vi "Main.vi"(11 "Module Admin":refnum<class "Delacor_lib_QMH_Module Admin.lvclass">) -> ()   [LabVIEW 2020, in "Settings.lvlib"]
doc: "This template is based off of the Queued Message Handler design pattern and the Queued Message Handler project template that ships with LabVIEW.\n\nThe main difference is that the queue is private to this module and communication between modules is performed via Broadcast and Request events.\n\nRequest events are wrapped in public API methods and are handled in the Event Handling Loop (EHL) of this VI. Any module can register for Broadcast events sent by this module. The EHL generates messages based on user interface actions.\n\nThe Message Handling Loop (MHL) processes messages generated by the EHL, or by other messages. The messages are string values, so new messages can be added easily to the Message Cases case structure in the MHL. Each message cluster can also provide an optional value for Message Data, which is a variant that can be converted to whatever message-specific data is required.\n_____\nBased on Delacor QMH Project Template 6.0.0.89."
uses:
  Settings.lvlib
  <vilib>/Delacor/Delacor QMH/Libraries/Module Admin_class/Delacor_lib_QMH_Module Admin.lvclass
  typeSignal--cluster.ctl
  Module Data--cluster.ctl
  Stop Argument--cluster.ctl
  <vilib>/Delacor/Delacor QMH/Libraries/Message Queue_class/Delacor_lib_QMH_Message Queue.lvclass/Delacor_lib_QMH_Message Queue.ctl
  <vilib>/Delacor/Delacor QMH/Libraries/Module Admin_class/Delacor_lib_QMH_Module Admin.lvclass/Delacor_lib_QMH_Module Admin.ctl
  Add signal Argument--cluster.ctl
  Add Digital Signal Argument--cluster.ctl
  Complete Tarea Argument--cluster.ctl
  Delete table Argument--cluster.ctl
  Delete Digital table Argument--cluster.ctl
  Delete All Table Argument--cluster.ctl
  Cancel Argument--cluster.ctl
  Type Signal loaded form database Argument--cluster.ctl
  <vilib>/Utility/miscctls.llb/LVPointTypeDef.ctl
  <vilib>/Delacor/Delacor QMH/Libraries/Message Queue_class/Delacor_lib_QMH_Enqueue Message (Single).vi
  <vilib>/Delacor/Delacor QMH/Libraries/Module Admin_class/Delacor_lib_QMH_Get External Launch.vi
  <vilib>/Utility/error.llb/Error Cluster From Error Code.vi
  <vilib>/ErrorRing/Error Ring.xnode
  <vilib>/Delacor/Delacor QMH/Libraries/Message Queue_class/Delacor_lib_QMH_Message Queue.lvclass
panel:
  in  "Tarea Lista":bool
  in  "Tab Control":enum32{"Page 1", "Page 2"}(tab)
  in  "Agregar Tarea":bool
  in  "Borrar una Tarea":bool
  in  "Analog Signal":T1={"DAQ Board Name"="DAQ_Simu1", "Analogicos Canales"=["DAQ_Simu1/ai1", "DAQ_Simu1/ai2"], "Port Digitales"=[], "Tiempo"=100.0, "number of samples "=1000, "rate"=1000.0, "Type"=enum."Analogico"}
  in  "Digital Signal":T1={"DAQ Board Name"="DAQ_Simu1", "Analogicos Canales"=["DAQ_Simu1/ai1", "DAQ_Simu1/ai2"], "Port Digitales"=[], "Tiempo"=100.0, "number of samples "=1000, "rate"=1000.0, "Type"=enum."Analogico"}
  in  "Borrar una Tarea Digital":bool
  in  "Agregar Tarea Digital":bool
  in  "Borrar todo":bool
  in  "Cancel Button":bool
  in  "Nombre de la Prueba":string
  out "error out":errorcluster
  out "Status":string
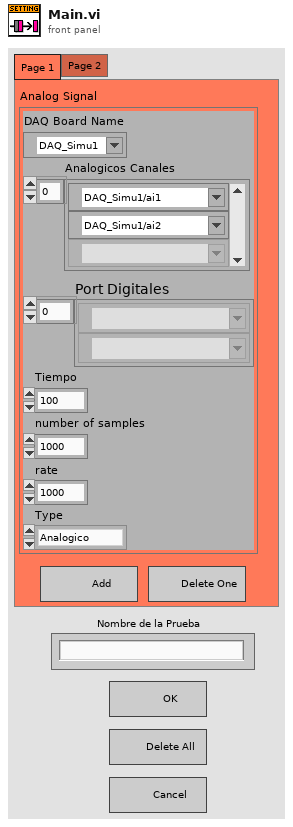
[diagram p1: front panel]
types:
  T1 = typedef "typeSignal--cluster.ctl" = cluster{"DAQ Board Name":tag, "Analogicos Canales":tag[], "Port Digitales":tag[], "Tiempo":dbl, "number of samples ":i32, "rate":dbl, "Type":enum16{"Analogico", "Digital"}}
  T2 = typedef "Settings.lvlib/Request Events--cluster.ctl" = cluster{"Stop Module":refnum<user-event>, "Show Panel":refnum<user-event>, "Hide Panel":refnum<user-event>, "Get Module Execution Status":refnum<user-event>, "Show Diagram":refnum<user-event>, "Add signal":refnum<user-event>, "Delete table":refnum<user-event>, "Cancel":refnum<user-event>, "Type Signal loaded form database":refnum<user-event>, "Delete All Table":refnum<user-event>, "Add Digital Signal":refnum<user-event>, "Delete Digital table":refnum<user-event>, "Complete Tarea":refnum<user-event>}
  T3 = typedef "Settings.lvlib/Module Data--cluster.ctl" = cluster{"Status":string, "Type Signal":T1, "Nombre de la Prueba":string}
  T4 = enum32{"invalid lock state", "Not Locked", "Locked (No Password)", "Password-protected"}
  T5 = typedef "Settings.lvlib/Stop Argument--cluster.ctl" = cluster{"Origin":string, "Exit via Stop Module Req?":bool, "Wait for Module to stop?":bool}
  T6 = typedef "Settings.lvlib/Add signal Argument--cluster.ctl" = cluster{"Agregar Tarea":bool}
  T7 = typedef "Settings.lvlib/Add Digital Signal Argument--cluster.ctl" = cluster{"Agregar Tarea Digital":bool}
  T8 = typedef "Settings.lvlib/Complete Tarea Argument--cluster.ctl" = cluster{"Tarea Lista":bool}
  T9 = typedef "Settings.lvlib/Delete table Argument--cluster.ctl" = cluster{"Borrar Tarea":bool}
  T10 = typedef "Settings.lvlib/Delete Digital table Argument--cluster.ctl" = cluster{"Borrar una Tarea Digital":bool}
  T11 = typedef "Settings.lvlib/Delete All Table Argument--cluster.ctl" = cluster{"Borrar todo":bool}
  T12 = typedef "Settings.lvlib/Cancel Argument--cluster.ctl" = cluster{"Cancel Button":bool}
  T13 = typedef "Settings.lvlib/Type Signal loaded form database Argument--cluster.ctl" = cluster{"Type Signal":T1, "Nombre de la Prueba":string}
  T14 = typedef "LVPointTypeDef.ctl" = cluster{"Horizontal":i16, "Vertical":i16}
  T15 = enum32{"Invalid", "Standard", "Closed", "Hidden", "Minimized", "Maximized"}
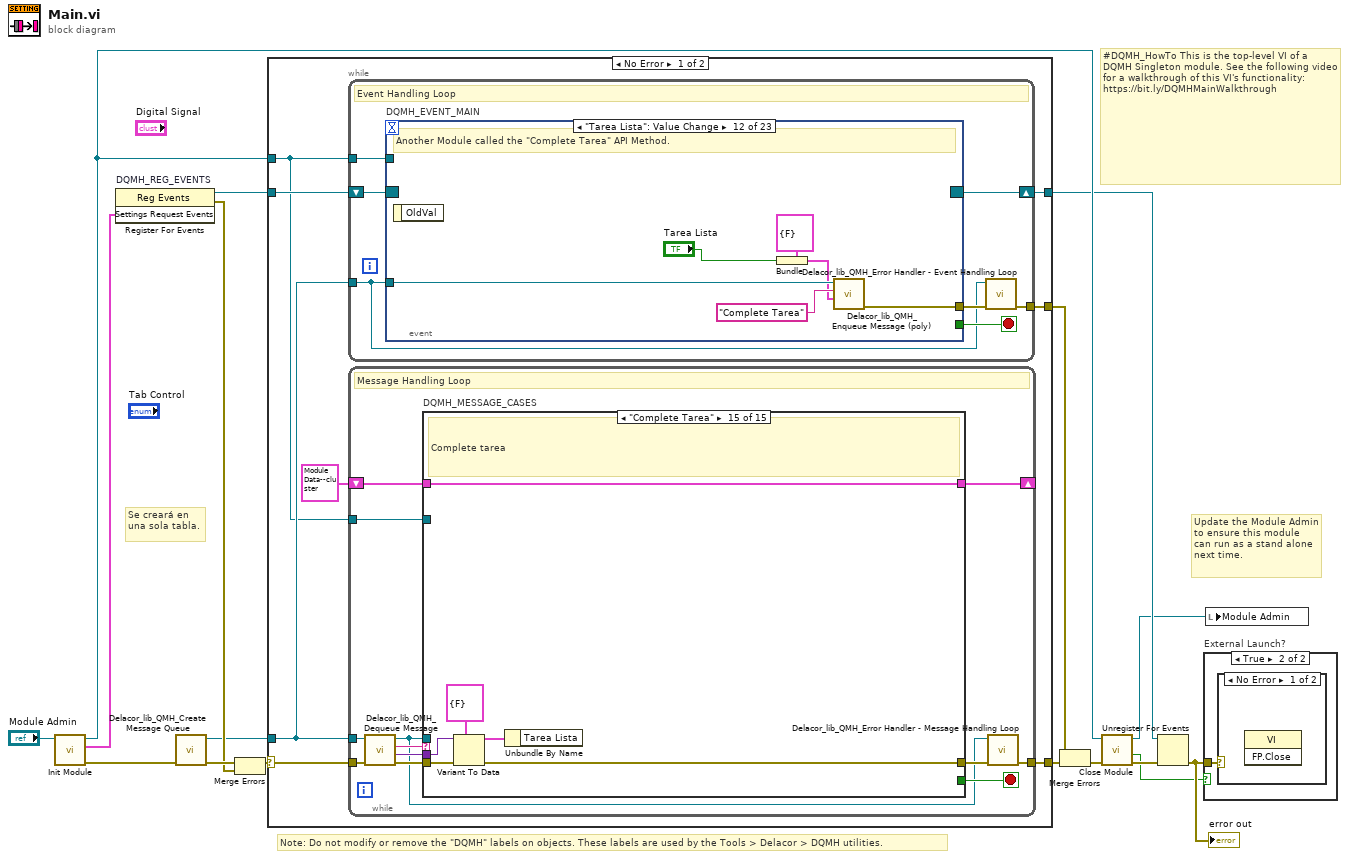
[diagram p0: block diagram]
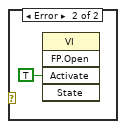
[diagram p3: hidden frame]
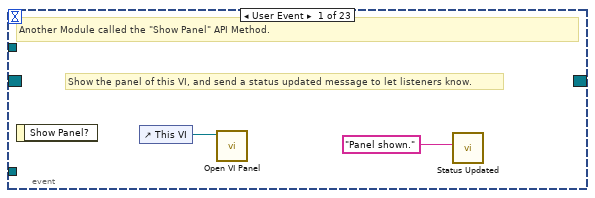
[diagram p4: hidden frame]
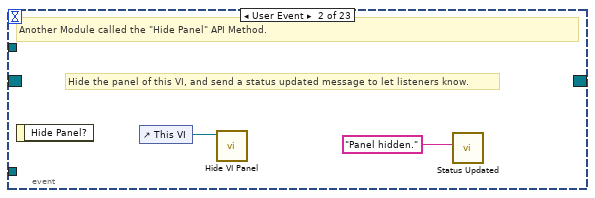
[diagram p5: hidden frame]
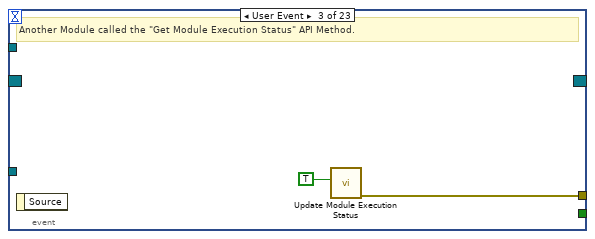
[diagram p6: hidden frame]
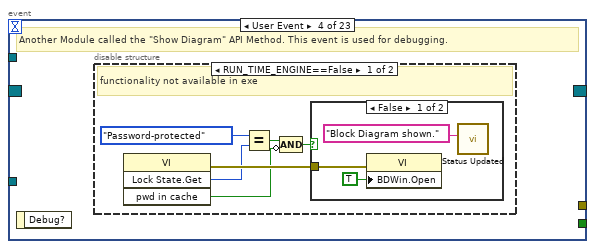
[diagram p7: hidden frame]
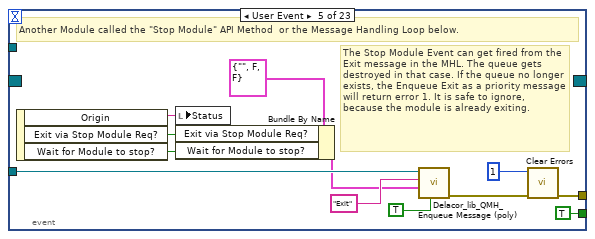
[diagram p10: hidden frame]
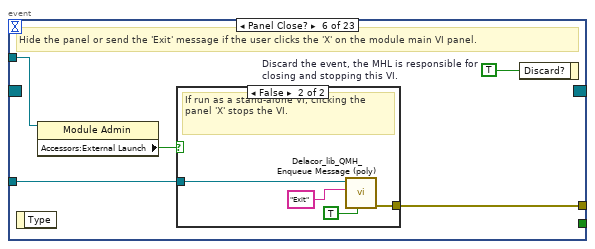
[diagram p11: hidden frame]
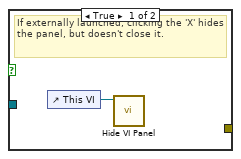
[diagram p12: hidden frame]
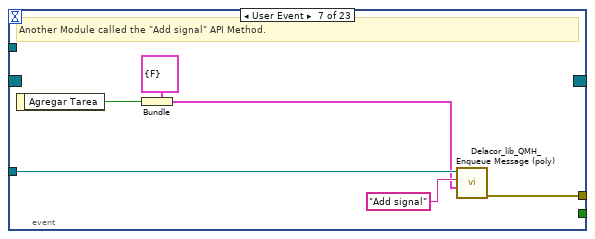
[diagram p13: hidden frame]
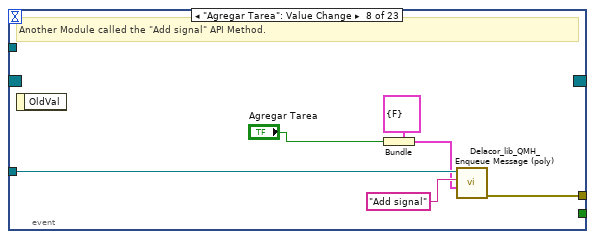
[diagram p14: hidden frame]
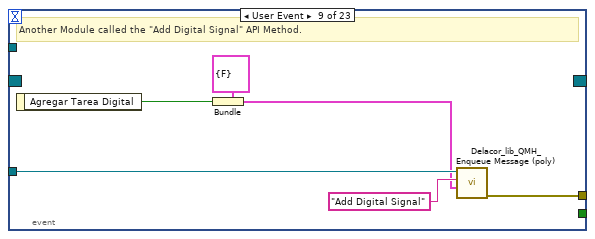
[diagram p15: hidden frame]
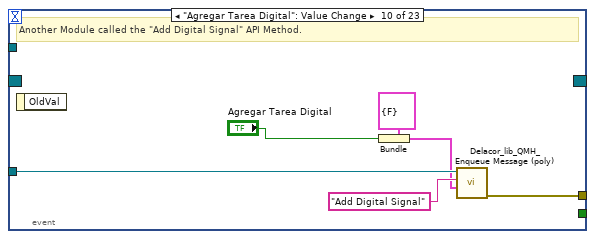
[diagram p16: hidden frame]
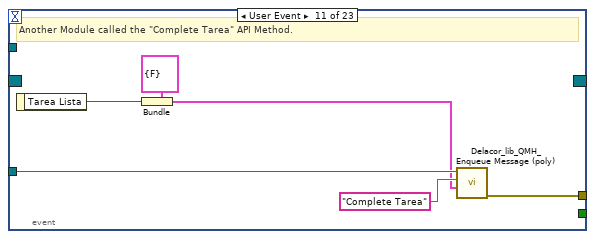
[diagram p17: hidden frame]
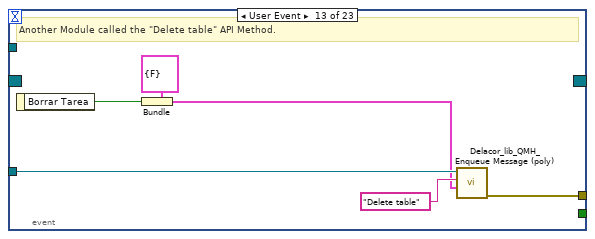
[diagram p18: hidden frame]
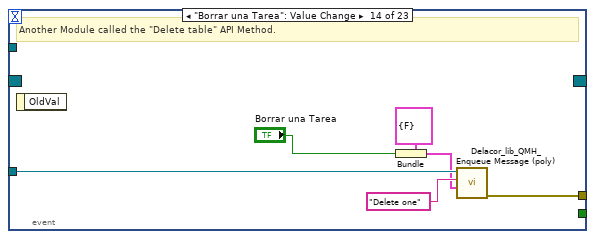
[diagram p19: hidden frame]
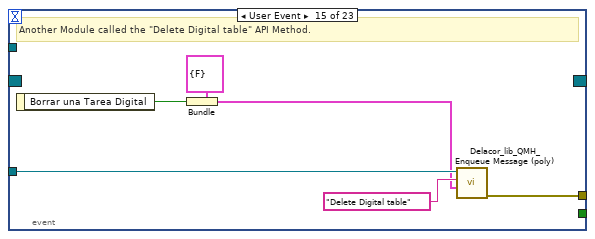
[diagram p20: hidden frame]
diagram:
  # "Se creará en una sola tabla."
  # "#DQMH_HowTo This is the top-level VI of a DQMH Singleton module. See the following video for a walkthrough of this VI's functionality: https://bit.ly/DQMHMainWalkthrough"
  # "Note: Do not modify or remove the \"DQMH\" labels on objects. These labels are used by the Tools > Delacor > DQMH utilities."
  # "Update the Module Admin to ensure this module can run as a stand alone next time."
  n1 = call "Init Module.vi"("Singleton Module Admin in"="Module Admin") -> ("error out"=w16:errorcluster, "Settings Request Events"=w5:T2, "Singleton Module Admin out"=w8:refnum<class "Delacor_lib_QMH_Module Admin.lvclass">)  [unwired: 8 in]
  n2 = register-events "DQMH_REG_EVENTS"(w5) -> (reference out=w6:refnum<event-registration>, error out=w9:errorcluster)  [unwired: 2 in]
  n3 = call <vilib>:"Delacor_lib_QMH_Create Message Queue.vi"("error in"=w16) -> ("error out"=w11:errorcluster, "Message Queue"=w4:refnum<class "Delacor_lib_QMH_Message Queue.lvclass">)  [unwired: 9 in]
  n4 = Merge Errors(w11, w9) -> (w10:errorcluster)
  n5 = case shown="No Error" w10 {
    selector: w10 -> [w23 w343]
    tunnel: [w25 w342] -> w17
    tunnel: [w22 w348] -> w7
    tunnel: w6 -> [w20 w348]
    tunnel: w4 -> [w19 w341]
    tunnel: [w24 _] -> w14
    tunnel: w8 -> [w18 w344]
    frame No Error {
      n6 = while {
        tunnel: w19 -> [w26]
        shift-right: [w29] -> w22
        shift-left: w20 -> [w30]
        tunnel: [w31] -> w24
        tunnel: w18 -> [w27]
        stop <- w28 stop-if-true
        # "Event Handling Loop"
        n7 = event "DQMH_EVENT_MAIN" shown="[11] \"Tarea Lista\": Value Change" {
          selector: w30 -> [_ _ _ _ _ _ _ _ _ _ _ _ _ _ _ _ _ _ _ _ _ _ _]
          dyn-events: [_ _ _ _ _ _ _ _ _ _ _ _ _ _ _ _ _ _ _ _ _ _ _] -> w29
          timeout: _ -> [_ _ _ _ _ _ _ _ _ _ _ _ _ _ _ _ _ _ _ _ _ _ _]
          tunnel: [_ _ _ _ TRUE ("Discard?") _ _ _ _ _ _ _ _ _ _ _ _ _ _ _ _ _ _] -> w28
          tunnel: w26 -> [_ _ _ _ w55 w62 w75 w81 w87 w93 w99 w105 w111 w117 w123 w129 w135 w141 w147 w153 w157 w161 w168]
          tunnel: [_ _ w38 _ w58 w64 w70 w77 w82 w89 w94 w101 w106 w113 w118 w125 w130 w137 w142 w149 w156 w160 w162] -> w32
          tunnel: w27 -> [_ _ _ _ _ w61 _ _ _ _ _ _ _ _ _ _ _ _ _ _ _ _ _]
          event User Event {
            # "Show the panel of this VI, and send a status updated message to let listeners know."
            # "Another Module called the \"Show Panel\" API Method."
            n8 = event-data() -> ()  [unwired: 1 in, 1 out]
            n9 = control-ref of="This VI"() -> (w34:refnum<vi>)
            n10 = call "Open VI Panel.vi"("VI"=w34) -> ()  [unwired: 10 in, 1 out]
            n11 = call "Status Updated.vi"("Status"="Panel shown." ("format string")) -> ()  [unwired: 10 in, 1 out]
          }
          event User Event {
            # "Hide the panel of this VI, and send a status updated message to let listeners know."
            # "Another Module called the \"Hide Panel\" API Method."
            n12 = event-data() -> ()  [unwired: 1 in, 1 out]
            n13 = control-ref of="This VI"() -> (w36:refnum<vi>)
            n14 = call "Hide VI Panel.vi"("VI"=w36) -> ()  [unwired: 10 in, 1 out]
            n15 = call "Status Updated.vi"("Status"="Panel hidden." ("format string")) -> ()  [unwired: 10 in, 1 out]
          }
          event User Event {
            # "Another Module called the \"Get Module Execution Status\" API Method."
            n16 = event-data() -> ()  [unwired: 1 in, 1 out]
            n17 = call "Update Module Execution Status.vi"("Running?"=TRUE) -> ("error out"=w38:errorcluster)  [unwired: 10 in]
          }
          event User Event {
            # "Another Module called the \"Show Diagram\" API Method. This event is used for debugging."
            n18 = event-data() -> ()  [unwired: 1 in, 1 out]
            n19 = disable-structure shown="RUN_TIME_ENGINE==False" {
              frame condition #0 (active) {
                # "functionality not available in exe"
                n20 = invoke class="VI" method="Lock State.Get"() -> (error out=w44:errorcluster, "Get Lock State"=w43:T4, "pwd in cache"=w40:bool)  [unwired: 4 in, 1 out]
                n21 = Equal?(x=T4."Password-protected", y=w43) -> (x = y?=w41:bool)
                n22 = Compound Arithmetic op=AND(w41, invert w40) -> (w39:bool)
                n23 = case shown="False" w39 {
                  tunnel: w44 -> [w47 _]
                  frame False {
                    n24 = property class="VI"(error in=w47, "BDWin.Open"=TRUE ("Block Diagram Window:Open")) -> ()  [unwired: 1 in, 2 out]
                    n25 = call "Status Updated.vi"("Status"="Block Diagram shown." ("format string")) -> ()  [unwired: 10 in, 1 out]
                  }
                  frame True {
                    # "Password-protected VI, and the password is not in the cache. Do not show the diagram."
                  }
                }
              }
              frame condition #1 {
              }
            }
          }
          event User Event {
            # "The Stop Module Event can get fired from the Exit message in the MHL. The queue gets destroyed in that case. If the queue no longer exists, the Enqueue Exit as a priority message will return error 1. It is safe to ignore, because the module is already exiting."
            # "Another Module called the \"Stop Module\" API Method  or the Message Handling Loop below."
            n26 = event-data() -> ("Origin"=w54:string, "Exit via Stop Module Req?"=w50:bool, "Wait for Module to stop?"=w49:bool)  [unwired: 1 in]
            n27 = local write "Status"(w54) -> ()
            n28 = Bundle By Name(cluster=T5 {"Origin"="", "Exit via Stop Module Req?"=FALSE, "Wait for Module to stop?"=FALSE} ("Stop Argument"), "Exit via Stop Module Req?"=w50, "Wait for Module to stop?"=w49) -> (w48:T5)
            n29 = call-poly <vilib>:"Delacor_lib_QMH_Enqueue Message (poly).vi"("Priority Message? (F)"=TRUE, "Message Data"=w48, "Message"="Exit", "Message Queue in"=w55) -> ("error out"=w59:errorcluster)  [unwired: 6 in, 1 out]
            n30 = call <vilib>:"Clear Errors.vi"("error in (no error)"=w59, "specific error code to clear (0: all)"=1) -> ("error out"=w58:errorcluster)  [unwired: 4 in, 1 out]
          }
          event Panel Close? {
            w63 = TRUE  # Discard the event, the MHL is responsible for closing and stopping this VI.
            # "Hide the panel or send the 'Exit' message if the user clicks the 'X' on the module main VI panel."
            n31 = event-data() -> ()  [unwired: 1 in, 1 out]
            n32 = property class="Module Admin"(reference=w61) -> ("Accessors:External Launch"=w60:bool)  [unwired: 1 in, 2 out]
            n33 = case shown="False" w60 {
              tunnel: w62 -> [_ w68]
              tunnel: [_ w69] -> w64
              frame True {
                # "If externally launched, clicking the 'X' hides the panel, but doesn't close it."
                n34 = control-ref of="This VI"() -> (w65:refnum<vi>)
                n35 = call "Hide VI Panel.vi"("VI"=w65) -> ()  [unwired: 10 in, 1 out]
              }
              frame False {
                # "If run as a stand-alone VI, clicking the panel 'X' stops the VI."
                n36 = call-poly <vilib>:"Delacor_lib_QMH_Enqueue Message (poly).vi"("Priority Message? (F)"=TRUE, "Message"="Exit", "Message Queue in"=w68) -> ("error out"=w69:errorcluster)  [unwired: 7 in, 1 out]
              }
            }
            n37 = event-data("Discard?"=w63) -> ()  [unwired: 1 in, 1 out]
          }
          event User Event {
            # "Another Module called the \"Add signal\" API Method."
            n38 = event-data() -> ("Agregar Tarea"=w71:bool)  [unwired: 1 in]
            n39 = Bundle(cluster=T6 {"Agregar Tarea"=FALSE} ("Add signal Argument"), "Agregar Tarea"=w71) -> (w72:T6)
            n40 = call-poly <vilib>:"Delacor_lib_QMH_Enqueue Message (poly).vi"("Message Data"=w72, "Message"="Add signal", "Message Queue in"=w75) -> ("error out"=w70:errorcluster)  [unwired: 7 in, 1 out]
          }
          event "Agregar Tarea": Value Change {
            # "Another Module called the \"Add signal\" API Method."
            n41 = event-data() -> ()  [unwired: 1 in, 1 out]
            n42 = Bundle(cluster=T6 {"Agregar Tarea"=FALSE} ("Add signal Argument"), "Agregar Tarea"="Agregar Tarea") -> (w78:T6)
            n43 = call-poly <vilib>:"Delacor_lib_QMH_Enqueue Message (poly).vi"("Message Data"=w78, "Message"="Add signal", "Message Queue in"=w81) -> ("error out"=w77:errorcluster)  [unwired: 7 in, 1 out]
          }
          event User Event {
            # "Another Module called the \"Add Digital Signal\" API Method."
            n44 = event-data() -> ("Agregar Tarea Digital"=w83:bool)  [unwired: 1 in]
            n45 = Bundle(cluster=T7 {"Agregar Tarea Digital"=FALSE} ("Add Digital Signal Argument"), "Agregar Tarea Digital"=w83) -> (w84:T7)
            n46 = call-poly <vilib>:"Delacor_lib_QMH_Enqueue Message (poly).vi"("Message Data"=w84, "Message"="Add Digital Signal", "Message Queue in"=w87) -> ("error out"=w82:errorcluster)  [unwired: 7 in, 1 out]
          }
          event "Agregar Tarea Digital": Value Change {
            # "Another Module called the \"Add Digital Signal\" API Method."
            n47 = event-data() -> ()  [unwired: 1 in, 1 out]
            n48 = Bundle(cluster=T7 {"Agregar Tarea Digital"=FALSE} ("Add Digital Signal Argument"), "Agregar Tarea Digital"="Agregar Tarea Digital") -> (w90:T7)
            n49 = call-poly <vilib>:"Delacor_lib_QMH_Enqueue Message (poly).vi"("Message Data"=w90, "Message"="Add Digital Signal", "Message Queue in"=w93) -> ("error out"=w89:errorcluster)  [unwired: 7 in, 1 out]
          }
          event User Event {
            # "Another Module called the \"Complete Tarea\" API Method."
            n50 = event-data() -> ("Tarea Lista"=w95:bool)  [unwired: 1 in]
            n51 = Bundle(cluster=T8 {"Tarea Lista"=FALSE} ("Complete Tarea Argument"), "Tarea Lista"=w95) -> (w96:T8)
            n52 = call-poly <vilib>:"Delacor_lib_QMH_Enqueue Message (poly).vi"("Message Data"=w96, "Message"="Complete Tarea", "Message Queue in"=w99) -> ("error out"=w94:errorcluster)  [unwired: 7 in, 1 out]
          }
          event "Tarea Lista": Value Change {
            # "Another Module called the \"Complete Tarea\" API Method."
            n53 = event-data() -> ()  [unwired: 1 in, 1 out]
            n54 = Bundle(cluster=T8 {"Tarea Lista"=FALSE} ("Complete Tarea Argument"), "Tarea Lista"="Tarea Lista") -> (w102:T8)
            n55 = call-poly <vilib>:"Delacor_lib_QMH_Enqueue Message (poly).vi"("Message Data"=w102, "Message"="Complete Tarea", "Message Queue in"=w105) -> ("error out"=w101:errorcluster)  [unwired: 7 in, 1 out]
          }
          event User Event {
            # "Another Module called the \"Delete table\" API Method."
            n56 = event-data() -> ("Borrar Tarea"=w107:bool)  [unwired: 1 in]
            n57 = Bundle(cluster=T9 {"Borrar Tarea"=FALSE} ("Delete table Argument"), "Borrar Tarea"=w107) -> (w108:T9)
            n58 = call-poly <vilib>:"Delacor_lib_QMH_Enqueue Message (poly).vi"("Message Data"=w108, "Message"="Delete table", "Message Queue in"=w111) -> ("error out"=w106:errorcluster)  [unwired: 7 in, 1 out]
          }
          event "Borrar una Tarea": Value Change {
            # "Another Module called the \"Delete table\" API Method."
            n59 = event-data() -> ()  [unwired: 1 in, 1 out]
            n60 = Bundle(cluster=T9 {"Borrar Tarea"=FALSE} ("Delete table Argument"), "Borrar Tarea"="Borrar una Tarea") -> (w114:T9)
            n61 = call-poly <vilib>:"Delacor_lib_QMH_Enqueue Message (poly).vi"("Message Data"=w114, "Message"="Delete one", "Message Queue in"=w117) -> ("error out"=w113:errorcluster)  [unwired: 7 in, 1 out]
          }
          event User Event {
            # "Another Module called the \"Delete Digital table\" API Method."
            n62 = event-data() -> ("Borrar una Tarea Digital"=w119:bool)  [unwired: 1 in]
            n63 = Bundle(cluster=T10 {"Borrar una Tarea Digital"=FALSE} ("Delete Digital table Argument"), "Borrar una Tarea Digital"=w119) -> (w120:T10)
            n64 = call-poly <vilib>:"Delacor_lib_QMH_Enqueue Message (poly).vi"("Message Data"=w120, "Message"="Delete Digital table", "Message Queue in"=w123) -> ("error out"=w118:errorcluster)  [unwired: 7 in, 1 out]
          }
          event "Borrar una Tarea Digital": Value Change {
            # "Another Module called the \"Delete Digital table\" API Method."
            n65 = event-data() -> ()  [unwired: 1 in, 1 out]
            n66 = Bundle(cluster=T10 {"Borrar una Tarea Digital"=FALSE} ("Delete Digital table Argument"), "Borrar una Tarea Digital"="Borrar una Tarea Digital") -> (w126:T10)
            n67 = call-poly <vilib>:"Delacor_lib_QMH_Enqueue Message (poly).vi"("Message Data"=w126, "Message"="Delete Digital table", "Message Queue in"=w129) -> ("error out"=w125:errorcluster)  [unwired: 7 in, 1 out]
          }
          event User Event {
            # "Another Module called the \"Delete All Table\" API Method."
            n68 = event-data() -> ("Borrar todo"=w131:bool)  [unwired: 1 in]
            n69 = Bundle(cluster=T11 {"Borrar todo"=FALSE} ("Delete All Table Argument"), "Borrar todo"=w131) -> (w132:T11)
            n70 = call-poly <vilib>:"Delacor_lib_QMH_Enqueue Message (poly).vi"("Message Data"=w132, "Message"="Delete All Table", "Message Queue in"=w135) -> ("error out"=w130:errorcluster)  [unwired: 7 in, 1 out]
          }
          event "Borrar todo": Value Change {
            # "Another Module called the \"Delete All Table\" API Method."
            n71 = event-data() -> ()  [unwired: 1 in, 1 out]
            n72 = Bundle(cluster=T11 {"Borrar todo"=FALSE} ("Delete All Table Argument"), "Borrar todo"="Borrar todo") -> (w138:T11)
            n73 = call-poly <vilib>:"Delacor_lib_QMH_Enqueue Message (poly).vi"("Message Data"=w138, "Message"="Delete All Table", "Message Queue in"=w141) -> ("error out"=w137:errorcluster)  [unwired: 7 in, 1 out]
          }
          event User Event {
            # "Another Module called the \"Cancel\" API Method."
            n74 = event-data() -> ("Cancel Button"=w143:bool)  [unwired: 1 in]
            n75 = Bundle(cluster=T12 {"Cancel Button"=FALSE} ("Cancel Argument"), "Cancel Button"=w143) -> (w144:T12)
            n76 = call-poly <vilib>:"Delacor_lib_QMH_Enqueue Message (poly).vi"("Message Data"=w144, "Message"="Cancel", "Message Queue in"=w147) -> ("error out"=w142:errorcluster)  [unwired: 7 in, 1 out]
          }
          event "Cancel Button": Value Change {
            # "Another Module called the \"Cancel\" API Method."
            n77 = event-data() -> ()  [unwired: 1 in, 1 out]
            n78 = Bundle(cluster=T12 {"Cancel Button"=FALSE} ("Cancel Argument"), "Cancel Button"="Cancel Button") -> (w150:T12)
            n79 = call-poly <vilib>:"Delacor_lib_QMH_Enqueue Message (poly).vi"("Message Data"=w150, "Message"="Cancel", "Message Queue in"=w153) -> ("error out"=w149:errorcluster)  [unwired: 7 in, 1 out]
          }
          event Value Change {
            n80 = event-data() -> ()  [unwired: 1 in, 1 out]
            n81 = call-poly <vilib>:"Delacor_lib_QMH_Enqueue Message (poly).vi"("Message Data"="Analog Signal", "Message"="Type Signal", "Message Queue in"=w157) -> ("error out"=w156:errorcluster)  [unwired: 7 in, 1 out]
          }
          event "Nombre de la Prueba": Value Change {
            n82 = event-data() -> ()  [unwired: 1 in, 1 out]
            n83 = call-poly <vilib>:"Delacor_lib_QMH_Enqueue Message (poly).vi"("Message Data"="Nombre de la Prueba", "Message"="Nombre Prueba", "Message Queue in"=w161) -> ("error out"=w160:errorcluster)  [unwired: 7 in, 1 out]
          }
          event User Event {
            # "Another Module called the \"Type Signal loaded form database\" API Method."
            n84 = event-data() -> ("Type Signal"=w164:T1, "Nombre de la Prueba"=w163:string)  [unwired: 1 in]
            n85 = Bundle(cluster=T13 {"Type Signal"={"DAQ Board Name"="DAQ_Simu1", "Analogicos Canales"=["DAQ_Simu1/ai1", "DAQ_Simu1/ai2"], "Port Digitales"=[], "Tiempo"=100.0, "number of samples "=1000, "rate"=1000.0, "Type"=enum."Analogico"}, "Nombre de la Prueba"=""} ("Type Signal loaded form database Argument"), "Type Signal"=w164, "Nombre de la Prueba"=w163) -> (w165:T13)
            n86 = call-poly <vilib>:"Delacor_lib_QMH_Enqueue Message (poly).vi"("Message Data"=w165, "Message"="Type Signal loaded form database", "Message Queue in"=w168) -> ("error out"=w162:errorcluster)  [unwired: 7 in, 1 out]
          }
        }
        n87 = call-dynamic "Delacor_lib_QMH_Error Handler - Event Handling Loop.vi"("error in"=w32, "Message Queue in"=w26) -> ("dup error in"=w31:errorcluster)  [unwired: 8 in, 1 out]
      }
      n88 = while {
        tunnel: w19 -> [w171]
        shift-right: [w175] -> _
        shift-left: T3 {"Status"="", "Type Signal"={"DAQ Board Name"="DAQ_Simu1", "Analogicos Canales"=["DAQ_Simu1/ai1", "DAQ_Simu1/ai2"], "Port Digitales"=[], "Tiempo"=100.0, "number of samples "=1000, "rate"=1000.0, "Type"=enum."Analogico"}, "Nombre de la Prueba"=""} ("Data Cluster") -> [w176]
        tunnel: w23 -> [w179]
        tunnel: [w177] -> w25
        tunnel: w18 -> [w169]
        stop <- w174 stop-if-true
        # "Message Handling Loop"
        n89 = call-dynamic "Delacor_lib_QMH_Dequeue Message.vi"("error in"=w179, "Message Queue in"=w171) -> ("error out"=w178:errorcluster, "Message Data"=w172:variant, "Message"=w173:string, "Message Queue out"=w170:refnum<class "Delacor_lib_QMH_Message Queue.lvclass">)  [unwired: 6 in]
        n90 = case "DQMH_MESSAGE_CASES" shown="\"Complete Tarea\"" w173 {
          selector: w173 -> [_ _ _ _ w250 _ _ _ _ _ _ _ _ _ _]
          tunnel: w170 -> [_ _ w220 w242 _ _ _ _ _ _ _ _ _ _ _]
          tunnel: w178 -> [w203 w210 w227 w248 w252 w273 w281 w289 w297 w304 w311 w322 w328 w334 w340]
          tunnel: [w202 w209 w223 w245 w253 w267 w275 w283 w291 w303 w310 w315 w326 w332 w338] -> w180
          tunnel: w176 -> [w193 w207 w222 w241 w251 w268 w280 w288 w296 w300 w308 w317 w327 w333 w339]
          tunnel: [w192 w207 w222 w241 w251 w268 w280 w288 w296 w298 w306 w316 w327 w333 w339] -> w175
          tunnel: [_ _ _ w240 _ _ _ _ _ _ _ _ _ _ _] -> w174
          tunnel: w172 -> [_ _ w221 w239 _ w271 w278 w286 w294 w302 w309 w320 w325 w331 w337]
          tunnel: w169 -> [w194 _ w219 w234 _ _ _ _ _ _ _ _ _ _ _]
          frame "Initialize" {
            w185 = "Initial Message" ("Initial Message")
            # "Si la tabla ya existe, leerla y\nrellenar los campos correspondientes"
            # "#Crear_Tabla_si_no_existe"
            # "Initialize - Any operation that needs to be done before the module can receive messages. Synchronize Caller Events.vi will inform Start Module.vi that the module has launched and is ready to receive messages. Module Did Init.vi will broadcast that the module initialized."
            n91 = call "Synchronize Caller Events.vi"("error in (no error)"=w203, "Singleton Module Admin in"=w194) -> ("error out"=w187:errorcluster, "Singleton Module Admin out"=w189:refnum<class "Delacor_lib_QMH_Module Admin.lvclass">)  [unwired: 8 in]
            n92 = property class="Module Admin"(reference=w189) -> ("Accessors:External Launch"=w198:bool)  [unwired: 1 in, 2 out]
            n93 = call "Create Table.vi"("error in (no error)"=w187) -> ("error out"=w186:errorcluster)  [unwired: 10 in]
            n94 = call "Read prueba.vi"("error in (no error)"=w186) -> ("error out"=w182:errorcluster, "num Prueba"=w181:string)  [unwired: 9 in]
            n95 = Select(t=T15."Hidden" ("State"), s=w198, f=T15."Standard" ("State")) -> (s? t:f=w195:T15)
            n96 = call "Read settings.vi"("error in (no error)"=w182) -> ("error out"=w183:errorcluster, "Type Signal"=w184:T1)  [unwired: 9 in]
            n97 = call "Module Name--constant.vi"() -> ("Module Name"=w201:string)  [unwired: 11 in]
            n98 = call "Type Signal loaded form database.vi"("Nombre de la Prueba"=w181, "Type Signal"=w184) -> ()  [unwired: 9 in, 1 out]
            n99 = property class="VI"("Front Panel.Title"=w201) -> (reference out=w200:refnum<vi>, error out=w205:errorcluster)  [unwired: 2 in]
            n100 = call "Module Name--constant.vi"() -> ("Module Name"=w190:string)  [unwired: 11 in]
            n101 = Bundle By Name(cluster=w193, "Nombre de la Prueba"=w181, "Type Signal"=w184, "Status"=w185) -> (w192:T3)
            n102 = invoke class="VI" method="FP.Open"(reference=w200, error in=w205, "State"=w195) -> (reference out=w199:refnum<vi>, error out=w204:errorcluster)  [unwired: 2 in, 3 out]
            n103 = call "Module Did Init.vi"("error in (no error)"=w183, "Initialized?"=TRUE, "Origin"=w190) -> ("error out"=w202:errorcluster)  [unwired: 8 in]
            n104 = invoke class="VI" method="FP.Center"(reference=w199, error in=w204) -> ()  [unwired: 1 in, 3 out]
            n105 = property on="Pane" class="Pane"("Origin"=T14 {"Horizontal"=0, "Vertical"=0}) -> ()  [unwired: 2 in, 2 out]
            "Status" <- w185
          }
          frame "Simulate MHL Error" {
            # "#DQMH_HowTo The 'Simulate MHL Error' button  illustrates how the MHL handles errors. This event is instructional in nature and can be removed."
            # "Simulate an error occurring at the MHL"
            n106 = call "Module Name--constant.vi"() -> ("Module Name"=w206:string)  [unwired: 11 in]
            n107 = xnode "Error Ring"("parameter 0"=w206) -> ("error out"=w208:errorcluster)
            n108 = Merge Errors(w210, w208) -> (w209:errorcluster)
          }
          frame "Error" {
            # "#CodeRecommended - If you ever change the name of this \"Error\" message, you'll need to update the name in the Check Loop Error.vi as well."
            # "#CodeRecommended - If the module is running in standalone mode (External Launch = FALSE), this code will pop up an error dialog and call the 'Exit' message if an error occurs. Add more fine-grained error handling here."
            # "Error - Check the error message data and respond accordingly. This message is sent by the \"Error Handler\" VIs at the end of each loop in this application."
            n109 = property class="Module Admin"(reference=w219) -> ("Accessors:External Launch"=w218:bool)  [unwired: 1 in, 2 out]
            n110 = Variant To Data(error in=w227, type=errorcluster {"status"=FALSE, "code"=0, "source"=""} ("error constant"), Variant=w221) -> (data=w228:errorcluster, error out=w225:errorcluster)
            n111 = call "Error Reported.vi"("Error"=w228) -> ()  [unwired: 10 in, 1 out]
            n112 = case shown="False" w218 {
              tunnel: [w233 _] -> w224
              tunnel: w220 -> [w231 _]
              tunnel: w228 -> [w232 _]
              frame False {
                # "If the module is running standalone, then pop up an error dialog and call the \"Exit\" message."
                n113 = call <vilib>:"Simple Error Handler.vi"("error in (no error)"=w232) -> ()  [unwired: 4 in, 5 out]
                n114 = call-poly <vilib>:"Delacor_lib_QMH_Enqueue Message (poly).vi"("Priority Message? (F)"=TRUE, "Message"="Exit", "Message Queue in"=w231) -> ("error out"=w233:errorcluster)  [unwired: 7 in, 1 out]
              }
              frame True {
                # "If the module was launched externally, calling the Error Reported broadcast VI is the only action performed by the \"Error\" message. The module's caller can then process the error appropriately."
              }
            }
            n115 = Merge Errors(w225, w224) -> (w223:errorcluster)
            n116 = local write "error out"(w223) -> ()
          }
          frame "Exit" {
            w238 = 91  # 91: not all Exit messages will have an argument
            w240 = TRUE  # Stop the VI
            # "Release the message queue reference"
            # "#CodeNeeded - Add any required cleanup code here"
            # "Exit - Exit the application."
            n117 = Variant To Data(error in=w248, type=T5 {"Origin"="", "Exit via Stop Module Req?"=FALSE, "Wait for Module to stop?"=FALSE} ("Stop Argument"), Variant=w239) -> (data=w236:T5, error out=w244:errorcluster)
            n118 = call <vilib>:"Clear Errors.vi"("error in (no error)"=w244, "specific error code to clear (0: all)"=w238) -> ("error out"=w247:errorcluster)  [unwired: 4 in, 1 out]
            n119 = control-ref of="This VI"() -> (w235:refnum<vi>)
            n120 = call-dynamic "Delacor_lib_QMH_Release Message Queue.vi"("error in"=w247, "Message Queue"=w242) -> ("error out"=w246:errorcluster)  [unwired: 9 in]
            n121 = call "Handle Exit.vi"("Stop Argument"=w236, "Admin in"=w234, "VI reference"=w235) -> ("error out"=w243:errorcluster)  [unwired: 7 in, 1 out]
            n122 = Merge Errors(w246, w243) -> (w245:errorcluster)
          }
          frame Default {
            # "'Default' case only runs if there is a message that isn't defined in any of the other cases.  Output a programming error."
            n123 = call "Module Name--constant.vi"() -> ("Module Name"=w249:string)  [unwired: 11 in]
            n124 = xnode "Error Ring"("parameter 0"=w250, "parameter 1"=w249) -> ("error out"=w254:errorcluster)
            n125 = Merge Errors(w252, w254) -> (w253:errorcluster)
          }
          frame "Add signal" {
            # "add a new signal"
            n126 = Variant To Data(error in=w273, type=T6 {"Agregar Tarea"=FALSE} ("Add signal Argument"), Variant=w271) -> (data=w269:T6, error out=w272:errorcluster)
            n127 = Unbundle By Name(w269) -> ()  [unwired: 1 out]
            n128 = Unbundle By Name(w268) -> ("Nombre de la Prueba"=w264:string, "Type Signal"=w266:T1)
            n129 = call "save settings.vi"("Type Signal"=w266) -> ("error out"=w265:errorcluster)  [unwired: 10 in]
            n130 = call "save prueba.vi"("Nombre de la Prueba"=w264) -> ("error out"=w263:errorcluster)  [unwired: 10 in]
            n131 = Merge Errors(w263, w265, w272) -> (w267:errorcluster)
          }
          frame "Delete one" {
            # "Delete the whole table."
            n132 = Variant To Data(error in=w281, type=T9 {"Borrar Tarea"=FALSE} ("Delete table Argument"), Variant=w278) -> (data=w276:T9, error out=w279:errorcluster)
            n133 = Unbundle By Name(w276) -> ()  [unwired: 1 out]
            n134 = call "delete one.vi"() -> ("error out"=w274:errorcluster)  [unwired: 11 in]
            n135 = Merge Errors(w274, w279) -> (w275:errorcluster)
          }
          frame "Delete All Table" {
            # "Delete all the table."
            n136 = Variant To Data(error in=w289, type=T11 {"Borrar todo"=FALSE} ("Delete All Table Argument"), Variant=w286) -> (data=w284:T11, error out=w287:errorcluster)
            n137 = Unbundle By Name(w284) -> ()  [unwired: 1 out]
            n138 = call "delete all.vi"() -> ("error out"=w282:errorcluster)  [unwired: 11 in]
            n139 = Merge Errors(w282, w287) -> (w283:errorcluster)
          }
          frame "Cancel" {
            # "Cancel the signal"
            n140 = Variant To Data(error in=w297, type=T12 {"Cancel Button"=FALSE} ("Cancel Argument"), Variant=w294) -> (data=w292:T12, error out=w295:errorcluster)
            n141 = Unbundle By Name(w292) -> ()  [unwired: 1 out]
            n142 = call "Hide Panel.vi"() -> ("error out"=w290:errorcluster)  [unwired: 11 in]
            n143 = Merge Errors(w290, w295) -> (w291:errorcluster)
          }
          frame "Type Signal" {
            n144 = Variant To Data(error in=w304, type=T1 {"DAQ Board Name"="DAQ_Simu1", "Analogicos Canales"=["DAQ_Simu1/ai1", "DAQ_Simu1/ai2"], "Port Digitales"=[], "Tiempo"=100.0, "number of samples "=1000, "rate"=1000.0, "Type"=enum."Analogico"} ("Type Signal"), Variant=w302) -> (data=w299:T1, error out=w303:errorcluster)
            n145 = Bundle By Name(cluster=w300, "Type Signal"=w299) -> (w298:T3)
          }
          frame "Nombre Prueba" {
            n146 = Variant To Data(error in=w311, type="", Variant=w309) -> (data=w307:string, error out=w310:errorcluster)
            n147 = Bundle By Name(cluster=w308, "Nombre de la Prueba"=w307) -> (w306:T3)
          }
          frame "Type Signal loaded form database" {
            # "Type signal was loaded from database"
            n148 = Variant To Data(error in=w322, type=T13 {"Type Signal"={"DAQ Board Name"="DAQ_Simu1", "Analogicos Canales"=["DAQ_Simu1/ai1", "DAQ_Simu1/ai2"], "Port Digitales"=[], "Tiempo"=100.0, "number of samples "=1000, "rate"=1000.0, "Type"=enum."Analogico"}, "Nombre de la Prueba"=""} ("Type Signal loaded form database Argument"), Variant=w320) -> (data=w318:T13, error out=w321:errorcluster)
            n149 = Unbundle By Name(w318) -> ("Type Signal"=w312:T1, "Nombre de la Prueba"=w313:string)
            n150 = Bundle By Name(cluster=w317, "Type Signal"=w312, "Nombre de la Prueba"=w313) -> (w316:T3)
            n151 = call "Config has been set.vi"("Type Signal"=w312, "Nombre de la Prueba"=w313) -> ("error out"=w314:errorcluster)  [unwired: 8 in]
            n152 = local write "Nombre de la Prueba"(w313) -> ()
            n153 = Merge Errors(w314, w321) -> (w315:errorcluster)
            n154 = local write "Analog Signal"(w312) -> ()
          }
          frame "Add Digital Signal" {
            # "Add digital signal."
            n155 = Variant To Data(error in=w328, type=T7 {"Agregar Tarea Digital"=FALSE} ("Add Digital Signal Argument"), Variant=w325) -> (data=w323:T7, error out=w326:errorcluster)
            n156 = Unbundle By Name(w323) -> ()  [unwired: 1 out]
          }
          frame "Delete Digital table" {
            # "delete digital table"
            n157 = Variant To Data(error in=w334, type=T10 {"Borrar una Tarea Digital"=FALSE} ("Delete Digital table Argument"), Variant=w331) -> (data=w329:T10, error out=w332:errorcluster)
            n158 = Unbundle By Name(w329) -> ()  [unwired: 1 out]
          }
          frame "Complete Tarea" {
            # "Complete tarea"
            n159 = Variant To Data(error in=w340, type=T8 {"Tarea Lista"=FALSE} ("Complete Tarea Argument"), Variant=w337) -> (data=w335:T8, error out=w338:errorcluster)
            n160 = Unbundle By Name(w335) -> ()  [unwired: 1 out]
          }
        }
        n161 = call-dynamic "Delacor_lib_QMH_Error Handler - Message Handling Loop.vi"("error in"=w180, "Message Queue in"=w170) -> ("dup error in"=w177:errorcluster)  [unwired: 8 in, 1 out]
      }
    }
    frame Error {
      # "Synchronize Caller Events.vi will inform Start Module.vi that the module has launched and will let the code calling Start Module.vi register for broadcasts and would permit the caller receive the broadcast that an error occurred at launch time."
      n162 = call-dynamic "Delacor_lib_QMH_Release Message Queue.vi"("error in"=w343, "Message Queue"=w341) -> ("error out"=w342:errorcluster)  [unwired: 9 in]
      n163 = call "Synchronize Caller Events.vi"("Singleton Module Admin in"=w344) -> ("error out"=w349:errorcluster)  [unwired: 9 in, 1 out]
      n164 = call "Module Name--constant.vi"() -> ("Module Name"=w347:string)  [unwired: 11 in]
      n165 = Format Into String(format string="An error occurred during initialization. %s is no longer running.", w347) -> (resulting string=w345:string)  [unwired: 2 in, 1 out]
      n166 = Merge Errors(w342, w349) -> (w350:errorcluster)
      n167 = call "Error Reported.vi"("Additional Information"=w345, "Error"=w350) -> ()  [unwired: 9 in, 1 out]
    }
  }
  n168 = Merge Errors(w14, w17) -> (w13:errorcluster)
  n169 = call "Close Module.vi"("error in (no error)"=w13, "Module Admin in"=w8) -> ("error out"=w15:errorcluster, "External Launch"=w1:bool, "Module Admin out"=w2:refnum<class "Delacor_lib_QMH_Module Admin.lvclass">)  [unwired: 7 in]
  n170 = Unregister For Events(event registration refnum=w7, error in=w15) -> (error out=w12:errorcluster)
  "error out" <- w12
  n171 = case "External Launch?" shown="True" w1 {
    tunnel: w12 -> [_ w351]
    frame False {
    }
    frame True {
      n172 = case shown="No Error" w351 {
        frame No Error {
          n173 = invoke class="VI" method="FP.Close"() -> ()  [unwired: 3 in, 3 out]
        }
        frame Error {
          n174 = invoke class="VI" method="FP.Open"("Activate"=TRUE ("Activate?")) -> ()  [unwired: 4 in, 5 out]
        }
      }
    }
  }
  n175 = local write "Module Admin"(w2) -> ()
